vi "Get Channel References.vi"(8 "error in":errorcluster, 11 "Section Ref in":T1 format="%.0x") -> (0 "error out":errorcluster, 2 "Output Data Channel Refs":T1[](array[typedef]) format="%.0x", 3 "Input Data Channel Refs":T1[](array[typedef]) format="%.0x")   [LabVIEW 2019, in "Software Multi-Plex System Explorer.lvlib"]
uses:
  Software Multi-Plex System Explorer.lvlib
  <vilib>/NI VeriStand/Custom Device API/Custom Device Item Ref.ctl
  Shared/Constants.vi
  <vilib>/NI VeriStand/Custom Device Tools/Custom Device Utility Library/NI VeriStand - Search for All Items by GUID.vi
  <vilib>/NI VeriStand/Custom Device Tools/Custom Device Utility Library/Custom Device Utility Library.lvlib
  Shared/Software Multi-Plex Shared.lvlib
  <vilib>/NI VeriStand/Custom Device API/Custom Device API.lvlib
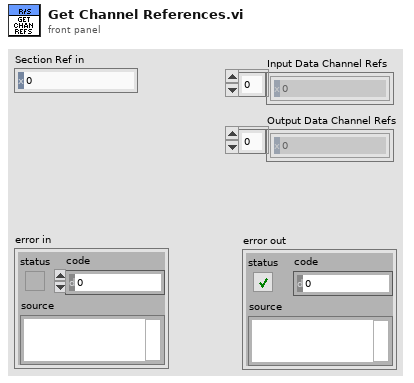
[diagram p1: front panel]
types:
  T1 = typedef "Custom Device API.lvlib/Custom Device Item Ref.ctl" = u64
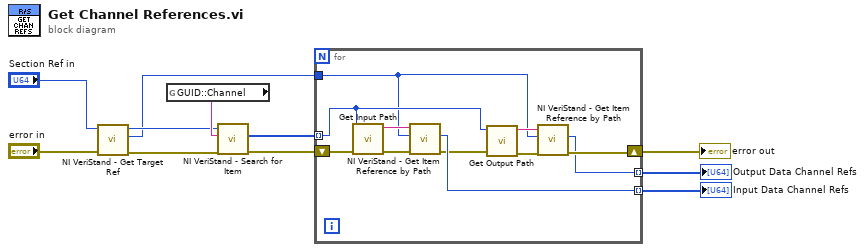
[diagram p0: block diagram]
diagram:
  n1 = call <vilib>:"NI VeriStand - Get Target Ref.vi"("error in"="error in", "Item Ref in"="Section Ref in") -> ("error out"=w4:errorcluster, "Target Ref"=w6:T1, "Item Ref out"=w7:T1)  [unwired: 6 in, 1 out]
  n2 = global read "Constants.vi" "GUID::Channel"() -> (w11:string)
  n3 = call-poly <vilib>:"NI VeriStand - Search for Item.vi"("error in"=w4, "Item GUID"=w11, "Section Ref in"=w7) -> ("error out"=w10:errorcluster, "Item Refs"=w9:T1[])  [unwired: 5 in, 2 out]
  n4 = for {
    shift-right: [w13] -> w3
    shift-left: w10 -> [w22]
    tunnel: w9 -> [w17] mode=indexing
    tunnel: w6 -> [w14]
    tunnel: [w19] -> w1 mode=indexing
    tunnel: [w12] -> w2 mode=indexing
    n5 = call "Get Input Path.vi"("error in (no error)"=w22, "Item Ref in"=w17) -> ("error out"=w21:errorcluster, "Input Path"=w20:string)  [unwired: 8 in]
    n6 = call <vilib>:"NI VeriStand - Get Item Reference by Path.vi"("error in (no error)"=w21, "Root Ref"=w14, "Item Path in"=w20) -> ("error out"=w18:errorcluster, "Item Ref"=w19:T1)  [unwired: 5 in, 2 out]
    n7 = call "Get Output Path.vi"("error in (no error)"=w18, "Item Ref in"=w17) -> ("error out"=w16:errorcluster, "Output Path"=w15:string)  [unwired: 7 in, 1 out]
    n8 = call <vilib>:"NI VeriStand - Get Item Reference by Path.vi"("error in (no error)"=w16, "Root Ref"=w14, "Item Path in"=w15) -> ("error out"=w13:errorcluster, "Item Ref"=w12:T1)  [unwired: 5 in, 2 out]
  }
  "error out" <- w3
  "Output Data Channel Refs" <- w2
  "Input Data Channel Refs" <- w1
